vi "Stop Animation.vi"(8 "Error In":errorcluster, 11 "Animation Config":T1) -> (0 "Error Out":errorcluster)   [LabVIEW 2011, in "LVH-Toolbox.lvlib" / "LVH-SystemTools.lvlib"]
uses:
  LVH-SystemTools.lvlib
  Private/UI/Animations/Animation Config.ctl
  <vilib>/picture/picture.llb/imagedata.ctl
  Private/UI/Type Defs/FGV States.ctl
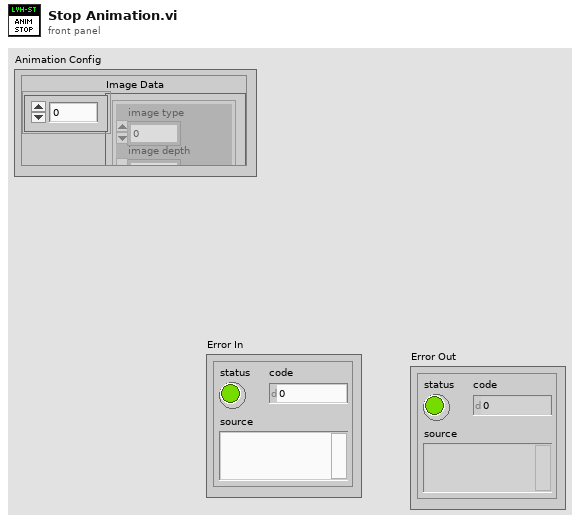
[diagram p1: front panel]
types:
  T1 = typedef "LVH-Toolbox.lvlib/LVH-SystemTools.lvlib/Animation Config.ctl" = cluster{"Image Data":T2[], "FPS":u32, "Position":cluster{"X":i16, "Y":i16}}
  T2 = typedef "imagedata.ctl" = cluster{"image type":i32, "image depth":i32, "image":u8[], "mask":u8[], "colors":u32[], "Rectangle":cluster{"left":i16, "top":i16, "right":i16, "bottom":i16}}
  T3 = typedef "LVH-Toolbox.lvlib/LVH-SystemTools.lvlib/FGV States.ctl" = enum16{"Init", "Set", "Get"}
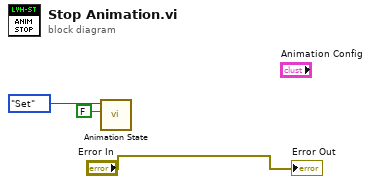
[diagram p0: block diagram]
diagram:
  n1 = call "Animation State.vi"("Running?"=FALSE, "Function"=FGV_States."Set") -> ()  [unwired: 9 in, 1 out]
  "Error Out" <- "Error In"
